vi "Determine Report Value.vi"(8 "error in (no error)":errorcluster, 10 "Value":string, 11 "U1 Data In":T1={"System Log"="", "[Array Of Threshold Refs]"=[], "[Array Of Boarder Refs]"=[], "APU Type"="", "APU Setup File"={"Sensor Info"=[], "Variables"=[], "CMM Table 106"=[], "CMM Table 106B "=[], "Accel Config"=[], "Report Sheet 1"=[], "Report Sheet 2"=[], "Report Sheet 3"=[]}, "ActiveValuetoRecordRow"=[], "ReportType"=[], "ReportValue"=[], "ActiveReportSheets"=[], "APUOn"=FALSE, "APUOnTime"=timestamp(0 s since 1904-01-01), "APUOffTime"=timestamp(0 s since 1904-01-01), "Recording"=FALSE, "Test Information"={"APU Part Number:"="555", "Model:"="5", "Serial Number:"="sad", "Customer:"="sad", "Work Order:"="asd", "Pre or Post SB"="Pre SB 49-7711", "Run Count"=0, "APU Selected"="<Select>"}, "APU RUN TIME"=timestamp(0 s since 1904-01-01)} {"APU RUN TIME" format="%<%H:%M:%S>T"; "Test Information"."Run Count" min=0 step=1; "APUOffTime" format="%<%x %.3X>T"; "APUOnTime" format="%<%x %.3X>T"}) -> (0 "error out":errorcluster, 3 "U1 Data out":T1={"System Log"="", "[Array Of Threshold Refs]"=[], "[Array Of Boarder Refs]"=[], "APU Type"="", "APU Setup File"={"Sensor Info"=[], "Variables"=[], "CMM Table 106"=[], "CMM Table 106B "=[], "Accel Config"=[], "Report Sheet 1"=[], "Report Sheet 2"=[], "Report Sheet 3"=[]}, "ActiveValuetoRecordRow"=[], "ReportType"=[], "ReportValue"=[], "ActiveReportSheets"=[], "APUOn"=FALSE, "APUOnTime"=timestamp(0 s since 1904-01-01), "APUOffTime"=timestamp(0 s since 1904-01-01), "Recording"=FALSE, "Test Information"={"APU Part Number:"="555", "Model:"="5", "Serial Number:"="sad", "Customer:"="sad", "Work Order:"="asd", "Pre or Post SB"="Pre SB 49-7711", "Run Count"=0, "APU Selected"="<Select>"}, "APU RUN TIME"=timestamp(0 s since 1904-01-01)} {"APU RUN TIME" format="%<%H:%M:%S>T"; "Test Information"."Run Count" min=0 step=1; "APUOffTime" format="%<%x %.3X>T"; "APUOnTime" format="%<%x %.3X>T"}, 4 "Reset Button Visable":bool=TRUE)   [LabVIEW 2018, in "Testing UI 1.lvlib"]
uses:
  Testing UI 1.lvlib
  Private Controls/UI 1 Data.ctl
  Top Level/Shared Controls/APU Setup File.ctl
  File IO/Public Controls/ReportType.ctl
  Controller (Host)/Public Controls/Test Information.ctl
  Controller (Host)/Public VIs/PreorPostSB.ctl
  Controller (Host)/Public Controls/APU Select.ctl
  Controller (Host)/Controller (Host).lvlib
  File IO/File IO.lvlib
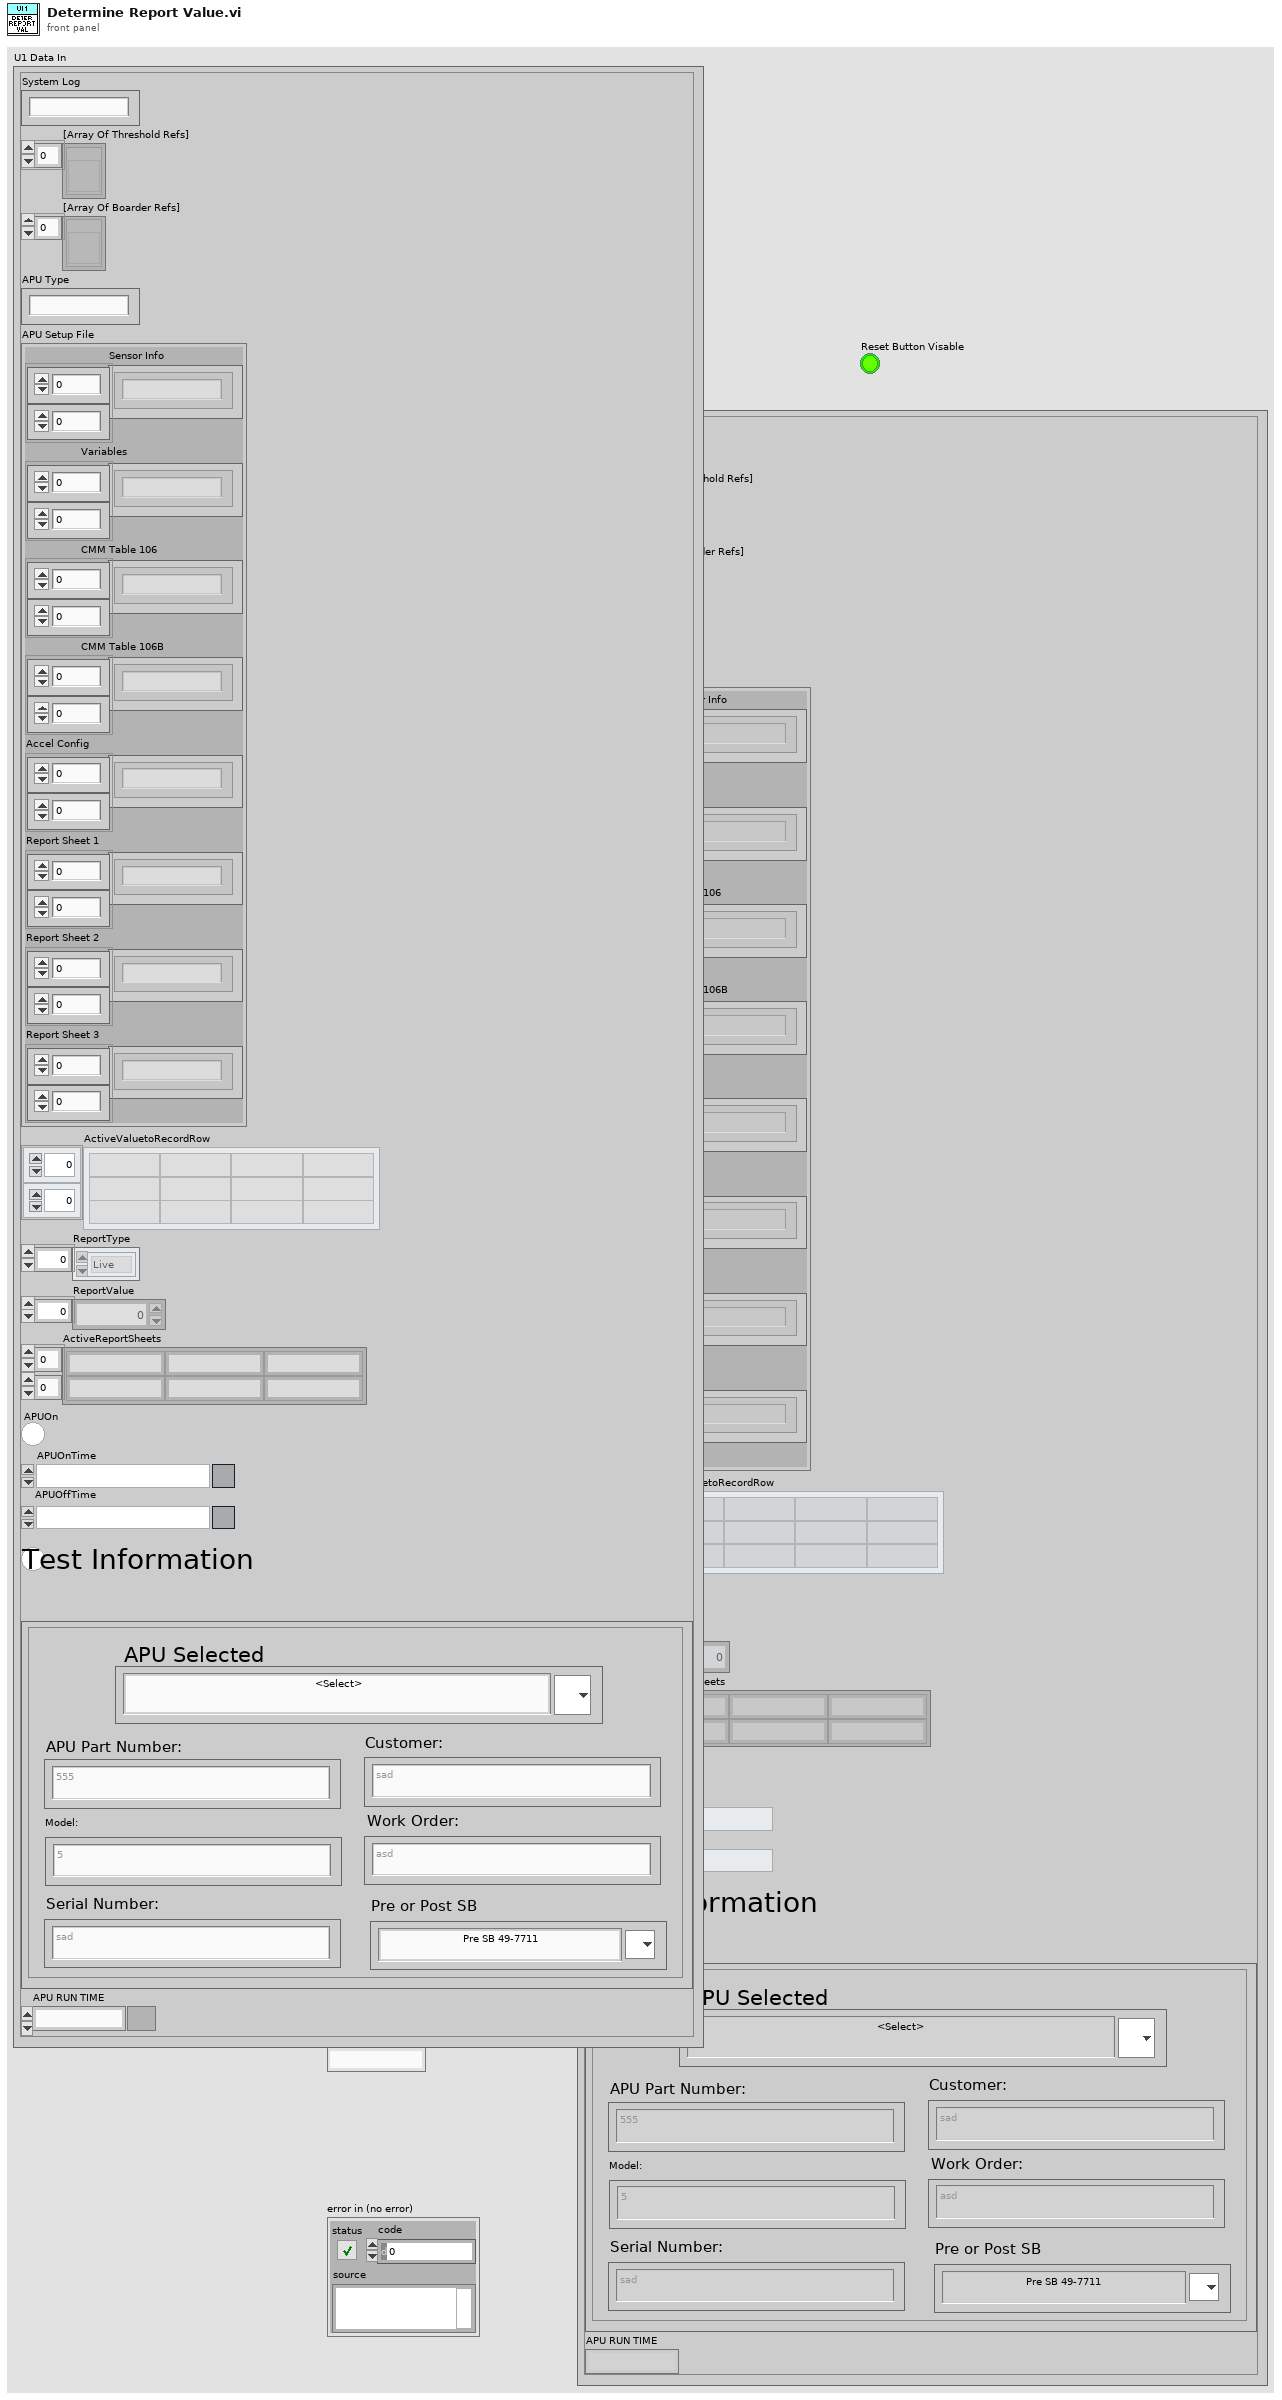
[diagram p1: front panel]
types:
  T1 = typedef "Testing UI 1.lvlib/UI 1 Data.ctl" = cluster{"System Log":string, "[Array Of Threshold Refs]":refnum<vi>[], "[Array Of Boarder Refs]":refnum<vi>[], "APU Type":string, "APU Setup File":T2, "ActiveValuetoRecordRow":string[][], "ReportType":T3[], "ReportValue":dbl[], "ActiveReportSheets":string[][], "APUOn":bool, "APUOnTime":timestamp, "APUOffTime":timestamp, "Recording":bool, "Test Information":T4, "APU RUN TIME":timestamp}
  T2 = typedef "APU Setup File.ctl" = cluster{"Sensor Info":string[][], "Variables":string[][], "CMM Table 106":string[][], "CMM Table 106B ":string[][], "Accel Config":string[][], "Report Sheet 1":string[][], "Report Sheet 2":string[][], "Report Sheet 3":string[][]}
  T3 = typedef "File IO.lvlib/ReportType.ctl" = enum16{"Live", "Min", "Max", "Deviation"}
  T4 = typedef "Controller (Host).lvlib/Test Information.ctl" = cluster{"APU Part Number:":string, "Model:":string, "Serial Number:":string, "Customer:":string, "Work Order:":string, "Pre or Post SB":T5, "Run Count":i32, "APU Selected":T6}
  T5 = typedef "Controller (Host).lvlib/PreorPostSB.ctl" = string
  T6 = typedef "Controller (Host).lvlib/APU Select.ctl" = string
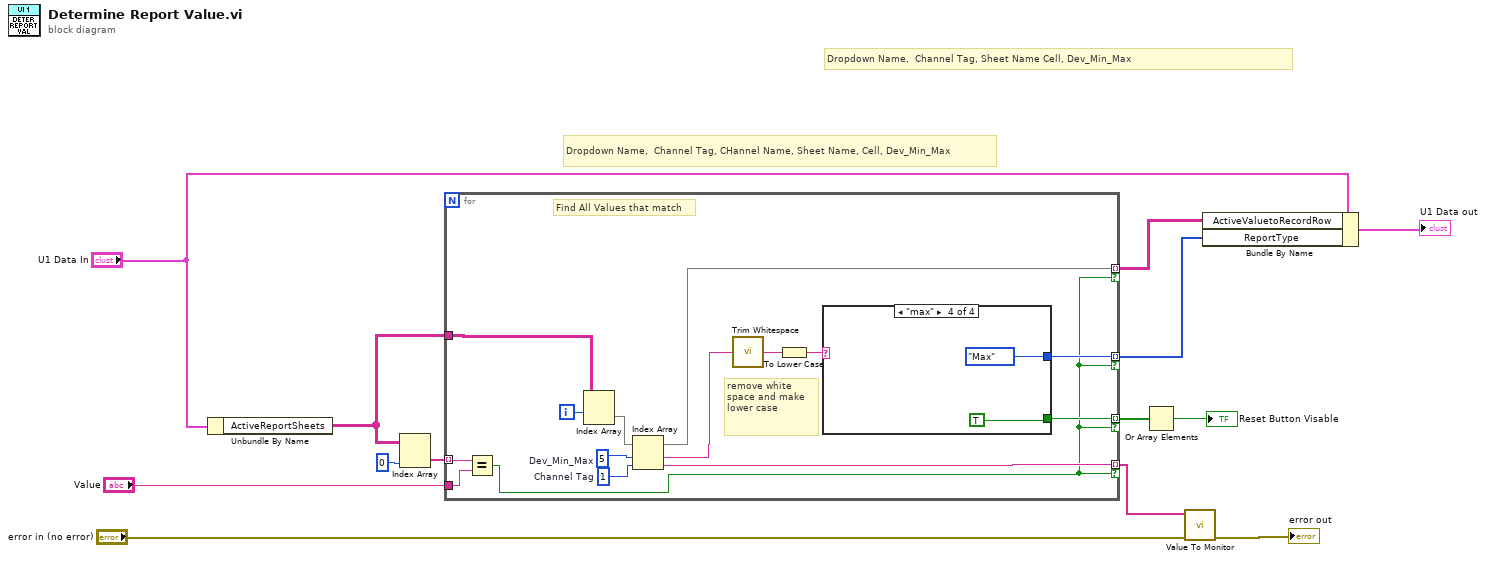
[diagram p0: block diagram]
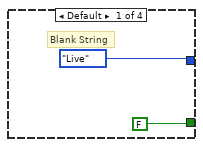
[diagram p2: hidden frame]
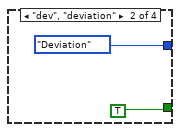
[diagram p3: hidden frame]
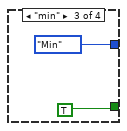
[diagram p4: hidden frame]
diagram:
  # "Dropdown Name,\t Channel Tag, CHannel Name,\tSheet Name, Cell, Dev_Min_Max"
  # "Dropdown Name,\t Channel Tag,\tSheet Name Cell, Dev_Min_Max"
  n1 = Unbundle By Name("U1 Data In") -> ("ActiveReportSheets"=w1:string[][])
  n2 = Index Array(array=w1, index (col)=0 ("disabled index (col)")) -> (element=w6:string[])  [unwired: 1 in]
  n3 = for {
    tunnel: [w27] -> w13 mode=indexing if=w14
    tunnel: [w26] -> w12 mode=indexing if=w14
    tunnel: w1 -> [w24]
    tunnel: w6 -> [w20] mode=indexing
    tunnel: "Value" -> [w19]
    tunnel: [w16] -> w4 mode=indexing if=w14
    tunnel: [w15] -> w3 mode=indexing if=w14
    i -> [w18]
    w25 = 1  # Channel Tag
    w23 = 5  # Dev_Min_Max
    # "Find All Values that match"
    # "remove white space and make\nlower case"
    n4 = Equal?(x=w20, y=w19) -> (x = y?=w14:bool)
    n5 = Index Array(array=w24, index (row)=w18) -> (element=w27:string[])  [unwired: 1 in]
    n6 = Index Array(array=w27, index #1=w23, index #2=w25) -> (element #1=w22:string, element #2=w26:string)
    n7 = call <vilib>:"Trim Whitespace.vi"("string"=w22) -> ("trimmed string"=w21:string)  [unwired: 1 in]
    n8 = To Lower Case(string=w21) -> (all lower case string=w17:string)
    n9 = case shown="\"max\"" w17 {
      tunnel: [ReportType."Live" ("ReportType") ReportType."Deviation" ("ReportType") ReportType."Min" ("ReportType") ReportType."Max" ("ReportType")] -> w16
      tunnel: [FALSE TRUE TRUE TRUE] -> w15
      frame Default {
        # "Blank String"
      }
      frame "dev", "deviation" {
      }
      frame "min" {
      }
      frame "max" {
      }
    }
  }
  n10 = Or Array Elements(Boolean array=w3) -> (logical OR=→"Reset Button Visable":bool)
  n11 = call "Value To Monitor.vi"("error in (no error)"="error in (no error)", "ValuesToMonitor"=w12) -> ("error out"=→"error out":errorcluster)  [unwired: 9 in]
  n12 = Bundle By Name(cluster="U1 Data In", "ActiveValuetoRecordRow"=w13, "ReportType"=w4) -> (→"U1 Data out":T1)
